vi "Read Status.vi"(11 "channel":T1) -> (0 "Pending Write":i32[](array[numeric]), 1 "Pending Read":i32[](array[numeric]), 2 "Usage Ratio":dbl[](array[numeric]), 3 "Queued Count":i32[](array[numeric]), 4 "Closed?":bool, 5 "Updated":timestamp, 7 "Sequence":u32)   [LabVIEW 2020, in "Flex.lvlib"]
doc: "Does not return values from the channel but reads the status of the channel and reads the queue status for all the queues used with lossless readers. This endpoint does not return values from the channel, just the status."
uses:
  Flex.lvlib
  ))Channel.ctl
  Element.ctl
  ChannelOp.ctl
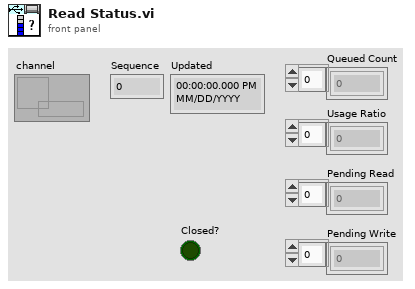
[diagram p1: front panel]
types:
  T1 = typedef "Flex.lvlib/))Channel.ctl" = refnum<queue>
  T2 = typedef "Flex.lvlib/ChannelOp.ctl" = enum16{"Get Refs", "Init", "Close", "Probe", "New Queue", "Remove Queue"}
  T3 = typedef "Flex.lvlib/Channel Data.ctl" = cluster{"Element":refnum<data-value>, "Queue Refs":refnum<data-value>, "Update":refnum<k4>}
  T4 = typedef "Flex.lvlib/Element Info.ctl" = cluster{"Value":T5, "Updated":timestamp, "Sequence":u32}
  T5 = typedef "Flex.lvlib/Element.ctl" = dbl
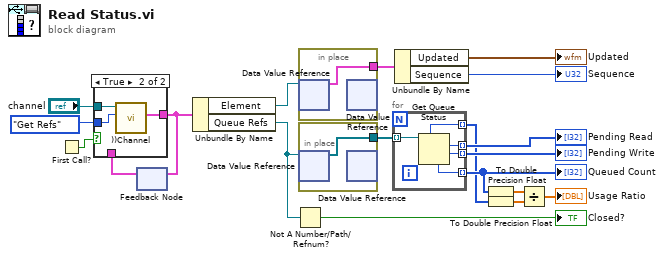
[diagram p0: block diagram]
diagram:
  n1 = First Call?() -> (First Call?: T/F=w18:bool)
  n2 = feedback #1() -> (w19:T3)  [unwired: 1 in]
  n3 = case shown="True" w18 {
    tunnel: w19 -> [w20 _]
    tunnel: [w20 w23] -> w15
    tunnel: "channel" -> [_ w22]
    tunnel: ChannelOp."Get Refs" ("channelOp") -> [_ w21]
    frame False {
    }
    frame True {
      n4 = call "))Channel.vi"("channelOp"=w21, "channel in"=w22) -> ("Channel Data"=w23:T3)  [unwired: 6 in, 3 out]
    }
  }
  n5 = feedback-in #1(w15) -> ()
  n6 = Unbundle By Name(w15) -> ("Element"=w14:refnum<data-value>, "Queue Refs"=w7:refnum<data-value>)
  n7 = Not A Number/Path/Refnum?(number/path/refnum=w7) -> (NaN/Path/Refnum?=→"Closed?":bool)
  n8 = in-place {
    in-place-border: [w24] -> w10
    n9 = in-place-dvr #2(w14) -> (w24:T4)  [unwired: 1 out]
    n10 = in-place-dvr #2() -> ()  [unwired: 1 in, 2 out]
  }
  n11 = in-place {
    in-place-border: [w25] -> w13
    n12 = in-place-dvr #3(w7) -> (w25:refnum<queue>[])  [unwired: 1 out]
    n13 = in-place-dvr #3() -> ()  [unwired: 1 in, 2 out]
  }
  n14 = for {
    tunnel: w13 -> [w30] mode=indexing
    tunnel: [w29] -> w5 mode=indexing
    tunnel: [w28] -> w12 mode=indexing
    tunnel: [w27] -> w11 mode=indexing
    tunnel: [w26] -> w4 mode=indexing
    n15 = Get Queue Status(queue=w30) -> (max queue size=w26:i32, # pending remove=w27:i32, # pending insert=w28:i32, # elements in queue=w29:i32)  [unwired: 2 in, 4 out]
  }
  "Queued Count" <- w5
  "Pending Write" <- w12
  "Pending Read" <- w11
  n16 = Unbundle By Name(w10) -> ("Updated"=→"Updated":timestamp, "Sequence"=→"Sequence":u32)
  n17 = To Double Precision Float(number=w5) -> (double precision float=w3:dbl[])
  n18 = To Double Precision Float(number=w4) -> (double precision float=w2:dbl[])
  n19 = Divide(x=w3, y=w2) -> (x/y=→"Usage Ratio":dbl[])
